vi "JX_GoHome.vi"(8 "error in (no error)":errorcluster, 10 "Axis":enum16{"X", "Y", "Z", "HOM"}(ring), 11 "Jiaxin_Stepper_Controller.lvlib:Jiaxin_Stepper.lvclass":refnum<class "Jiaxin_Stepper.lvclass">) -> (0 "error out":errorcluster, 3 "Jiaxin_Stepper_Controller.lvlib:Jiaxin_Stepper.lvclass":refnum<class "Jiaxin_Stepper.lvclass">)   [LabVIEW 2023, in "Jiaxin_Stepper_Controller.lvlib" / "Jiaxin_Stepper.lvclass"]
uses:
  Jiaxin_Stepper/Jiaxin_Stepper.lvclass
  UIs/TranslationStage_UI/TranslationStage_UI/StageMoveDone_For_UI.ctl
  Jiaxin_Stepper/Jiaxin_Stepper.lvclass/Jiaxin_Stepper.ctl
  <vilib>/ActorFramework/Actor/Actor.lvclass/Actor.ctl
  Interfaces/AbstractInstrumentClasses/TranslationStages_LV/TranslationStagesComm Messages/StageMoveDone Msg/StageMoveDone Msg.lvclass/StageMoveDone Msg.ctl
  <vilib>/ActorFramework/Message Enqueuer/Message Enqueuer.lvclass/Message Enqueuer.ctl
  <vilib>/ActorFramework/Message Enqueuer/Enqueue.vi
  Interfaces/AbstractInstrumentClasses/TranslationStages_LV/TranslationStagesComm Messages/StageMoveDone Msg/StageMoveDone Msg.lvclass
  <vilib>/ActorFramework/Message Priority Queue/Priority Enqueue.vi
  typedefs/typedefs.lvlib
  <vilib>/ActorFramework/Actor/Actor.lvclass
  C:/Program Files/National Instruments/LabVIEW 2023/vi.lib/ActorFramework/Actor/Actor.lvclass
  C:/Users/quantum/Documents/LVDAQ/ConcreteClasses/ConcreteInstrumentClasses/Jiaxin_Stepper_Controller/Jiaxin_Stepper/Jiaxin_Stepper.lvclass
  C:/Users/quantum/Documents/LVDAQ/Interfaces/InitDeinitInterface/InitDeinit/InitDeinit.lvclass
  C:/Users/quantum/Documents/LVDAQ/Interfaces/AbstractInstrumentClasses/TranslationStages_LV/TranslationStageInterface/TranslationStagesInterface.lvclass
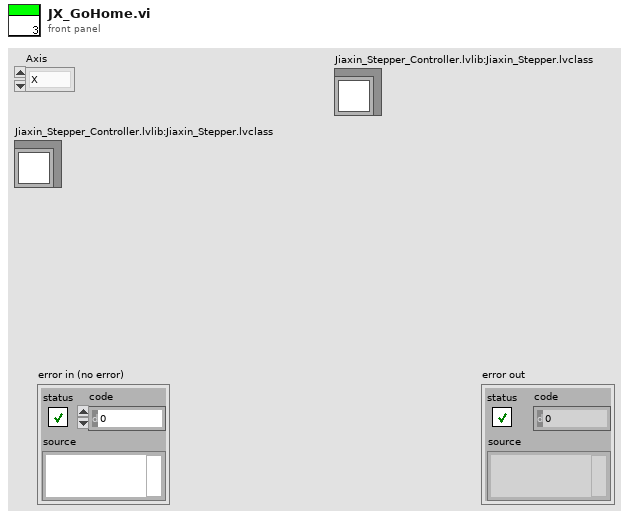
[diagram p1: front panel]
types:
  T1 = typedef "typedefs.lvlib/StageMoveDone_For_UI.ctl" = cluster{"CH1 Pos":sgl, "CH2 Pos":dbl, "CH3 Pos":dbl, "CH4 Pos":dbl, "Home?":bool}
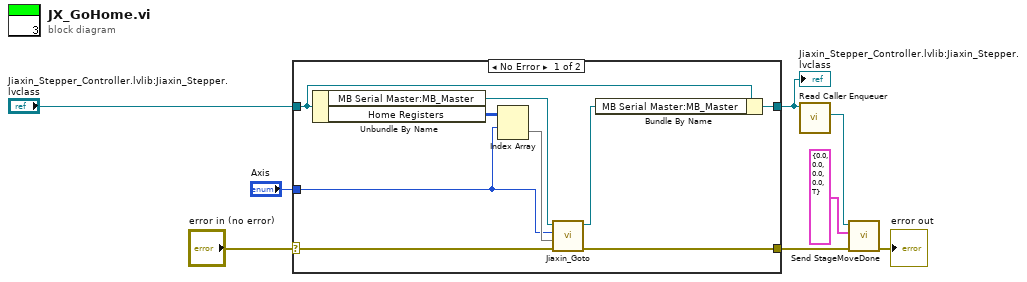
[diagram p0: block diagram]
diagram:
  n1 = case shown="No Error" "error in (no error)" {
    selector: "error in (no error)" -> [w13 w19]
    tunnel: [w12 w19] -> w2
    tunnel: [w16 w18] -> w4
    tunnel: "Jiaxin_Stepper_Controller.lvlib:Jiaxin_Stepper.lvclass" -> [w14 w18]
    tunnel: "Axis" -> [w9 _]
    frame No Error {
      n2 = Unbundle By Name(w14) -> ("MB Serial Master:MB_Master"=w15:refnum<class "MB_Master.lvclass">, "Home Registers"=w11:u16[][])
      n3 = Index Array(array=w11, index (row)=w9) -> (element=w10:u16[])  [unwired: 1 in]
      n4 = call "Jiaxin_Goto.vi"("error in (no error)"=w13, "Abs Position Registers"=w10, "Channel"=w9, "MB Serial Master:MB_Master"=w15) -> ("error out"=w12:errorcluster, "MB Serial Master:MB_Master"=w17:refnum<class "MB_Master.lvclass">)  [unwired: 6 in]
      n5 = Bundle By Name(cluster=w14, "MB Serial Master:MB_Master"=w17) -> (w16:refnum<class "Jiaxin_Stepper.lvclass">)
    }
    frame Error {
    }
  }
  "Jiaxin_Stepper_Controller.lvlib:Jiaxin_Stepper.lvclass" <- w4
  n6 = call <vilib>:"Read Caller Enqueuer.vi"("Actor"=w4) -> ("Caller Enqueuer"=w5:refnum<class "Message Enqueuer.lvclass">)  [unwired: 10 in]
  n7 = call "Send StageMoveDone.vi"("error in (no error)"=w2, "Positions"=T1 {"CH1 Pos"=0.0, "CH2 Pos"=0.0, "CH3 Pos"=0.0, "CH4 Pos"=0.0, "Home?"=TRUE}, "Message Enqueuer"=w5) -> ("error out"=→"error out":errorcluster)  [unwired: 7 in, 1 out]
